vi "tmp_toml_parse.vi"(8 "error in (no error)":errorcluster, 11 "text in":string) -> (0 "error out":errorcluster, 3 "sections":T1(array[cluster]))   [LabVIEW 2017]
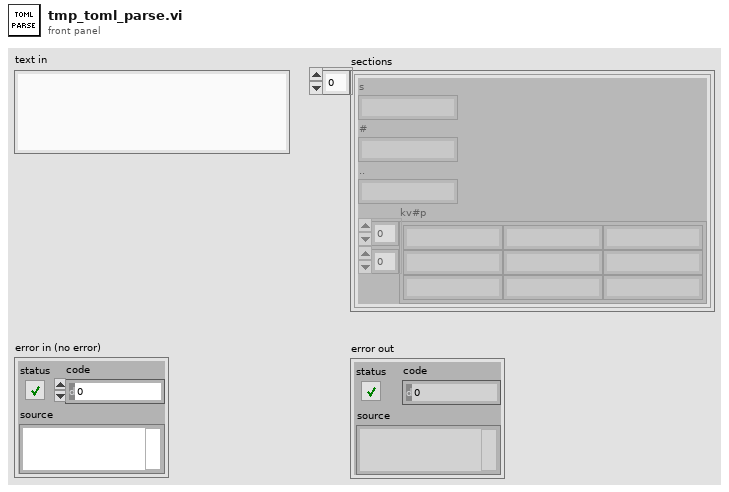
[diagram p1: front panel]
types:
  T1 = cluster{"s":string, "#":string, "..":string, "kv#p":string[][]}[]
  T2 = cluster{"s":string, "#":string, "..":string, "kv#p":string[][]}
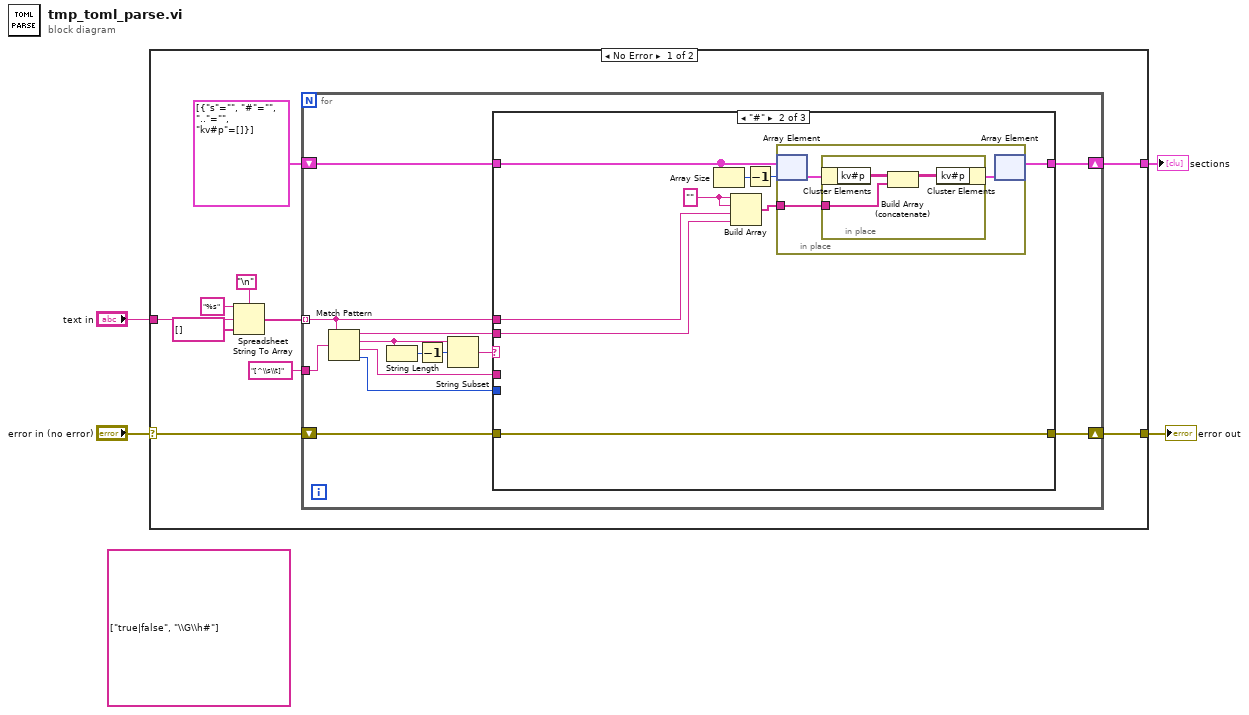
[diagram p0: block diagram]
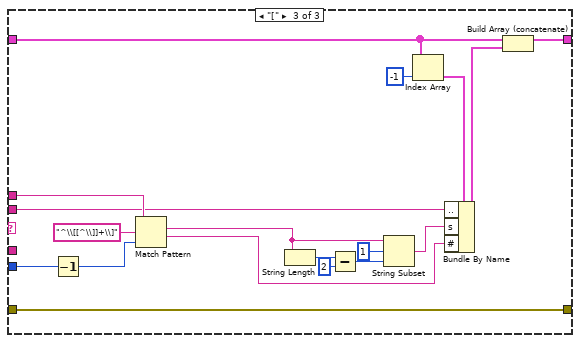
[diagram p3: hidden frame]
diagram:
  (unwired) string[] ["true|false", "\\G\\h#"]
  n1 = case shown="No Error" "error in (no error)" {
    selector: "error in (no error)" -> [w6 w63]
    tunnel: "text in" -> [w11 _]
    tunnel: [w7 _] -> w1
    tunnel: [w5 w63] -> w2
    frame No Error {
      n2 = Spreadsheet String To Array(delimiter (Tab)="\n", format string="%s", spreadsheet string=w11, array type (2D Dbl)=string[] []) -> (array=w10:string[])
      n3 = for {
        tunnel: w10 -> [w17] mode=indexing
        shift-right: [w22] -> w7
        shift-left: T1 [{"s"="", "#"="", ".."="", "kv#p"=[]}] ("sections 2") -> [w21]
        tunnel: "[^\\s\\t]" ("regular expression") -> [w27]
        shift-right: [w20] -> w5
        shift-left: w6 -> [w19]
        n4 = Match Pattern(string=w17, regular expression=w27) -> (before substring=w15:string, match substring=w26:string, after substring=w18:string, offset past match=w16:i32)  [unwired: 1 in]
        n5 = String Length(string=w26) -> (length=w25:i32)
        n6 = Decrement(x=w25) -> (x-1=w24:i32)
        n7 = String Subset(string=w26, offset (0)=w24) -> (substring=w23:string)  [unwired: 1 in]
        n8 = case shown="\"#\"" w23 {
          tunnel: [w29 w37 w59] -> w22
          tunnel: w21 -> [w29 w36 w50]
          tunnel: [w28 w38 w62] -> w20
          tunnel: w19 -> [w28 w38 w62]
          tunnel: w18 -> [_ _ _]
          tunnel: w17 -> [_ w32 w61]
          tunnel: w16 -> [_ _ w60]
          tunnel: w15 -> [_ w30 w47]
          frame "False", Default {
          }
          frame "#" {
            w33 = ""
            n9 = Array Size(array=w36) -> (size(s)=w35:i32)
            n10 = Build Array(w33, w33, w32, w30) -> (w31:string[])
            n11 = Decrement(x=w35) -> (x-1=w34:i32)
            n12 = in-place {
              in-place-border: w31 -> [w40]
              n13 = in-place-array #1(w36, w34) -> (w41:T2)
              n14 = in-place {
                in-place-border: w40 -> [w42]
                n15 = in-place-cluster #2(w41) -> ("kv#p"=w44:string[][])
                n16 = Build Array (concatenate)(w44, w42) -> (w43:string[][])
                n17 = in-place-cluster #2("kv#p"=w43) -> (w39:T2)
              }
              n18 = in-place-array #1(w39) -> (w37:T1)  [unwired: 1 out]
            }
          }
          frame "[" {
            n19 = Decrement(x=w60) -> (x-1=w57:i32)
            n20 = Match Pattern(string=w61, regular expression="^\\[[^\\]]+\\]", offset (0)=w57) -> (match substring=w56:string, after substring=w45:string)  [unwired: 2 out]
            n21 = String Length(string=w56) -> (length=w55:i32)
            n22 = Subtract(x=w55, y=2 ("x")) -> (x-y=w54:i32)
            n23 = String Subset(string=w56, offset (0)=1, length (rest)=w54) -> (substring=w46:string)
            n24 = Index Array(array=w50, index=-1) -> (element=w48:T2)
            n25 = Bundle By Name(cluster=w48, ".."=w47, "s"=w46, "#"=w45) -> (w51:T2)
            n26 = Build Array (concatenate)(w50, w51) -> (w59:T1)
          }
        }
      }
    }
    frame Error {
    }
  }
  "error out" <- w2
  "sections" <- w1
